vi "Pre Launch Init.vi"(11 "Test Manager in":refnum<class "Test Manager.lvclass">) -> (0 "error out":errorcluster, 3 "Test Manager out":refnum<class "Test Manager.lvclass">)   [LabVIEW 2020, in "Test Manager.lvlib" / "Test Manager.lvclass"]
doc: "Sends a high priority message to it's self to notify the monitor that it's spawned. If it's in the runtime environment, this message is never sent, meaning the monitor will never spawn\n\nCopyright: MGI\n\nAuthored by Derek Trepanier\nsupport@mooregoodideas.com\nwww.mooregoodideas.com\n\nCopyright (c) 2014, Moore Good Ideas, Inc.\n\nAll rights reserved.\n\nRedistribution and use in source and binary forms, with or without modification, are permitted provided that the following conditions are met:\n\n * Redistributions of source code must retain the above copyright notice, this list of conditions and the following disclaimer.\n * Redistributions in binary form must reproduce the above copyright notice, this list of conditions and the following disclaimer in the documentation and/or other materials provided with the distribution.\n * Neither the name of Moore Good Ideas, Inc. nor the names of its contributors may be used to endorse or promote products derived from this software without specific prior written permission.\n\nTHIS SOFTWARE IS PROVIDED BY THE COPYRIGHT HOLDERS AND CONTRIBUTORS \"AS IS\" AND ANY EXPRESS OR IMPLIED WARRANTIES, INCLUDING, BUT NOT LIMITED TO, THE IMPLIED WARRANTIES OF MERCHANTABILITY AND FITNESS FOR A PARTICULAR PURPOSE ARE DISCLAIMED. IN NO EVENT SHALL THE COPYRIGHT OWNER OR CONTRIBUTORS BE LIABLE FOR ANY DIRECT, INDIRECT, INCIDENTAL, SPECIAL, EXEMPLARY, OR CONSEQUENTIAL DAMAGES (INCLUDING, BUT NOT LIMITED TO, PROCUREMENT OF SUBSTITUTE GOODS OR SERVICES; LOSS OF USE, DATA, OR PROFITS; OR BUSINESS INTERRUPTION) HOWEVER CAUSED AND ON ANY THEORY OF LIABILITY, WHETHER IN CONTRACT, STRICT LIABILITY, OR TORT (INCLUDING NEGLIGENCE OR OTHERWISE) ARISING IN ANY WAY OUT OF THE USE OF THIS SOFTWARE, EVEN IF ADVISED OF THE POSSIBILITY OF SUCH DAMAGE."
uses:
  Test Manager.lvclass
  _Abstract Classes/Testing Asset/Testing Asset.lvclass
  _Abstract Classes/Test/Test.lvclass
  Test Manager.lvclass/Test Manager.ctl
  <vilib>/MGI/Monitored Actor/Monitored Actor/Monitored Actor/Monitored Actor.lvclass
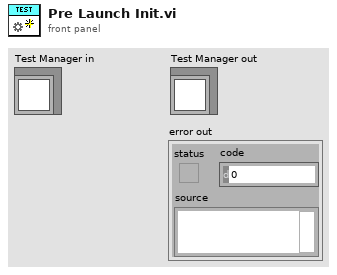
[diagram p1: front panel]
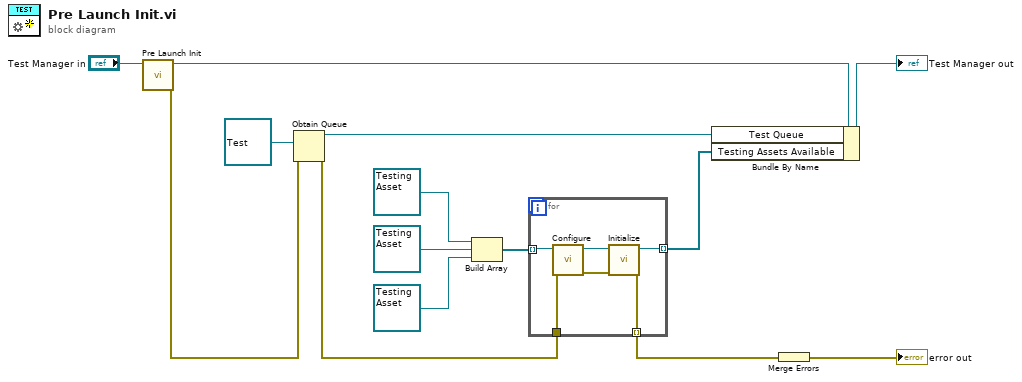
[diagram p0: block diagram]
diagram:
  n1 = call-parent "Pre Launch Init.vi"("Monitored Actor in"="Test Manager in") -> ("error out"=w10:errorcluster, "Monitored Actor out"=w12:refnum<class "Test Manager.lvclass">)  [unwired: 9 in]
  n2 = Obtain Queue(element data type=refnum<class "Test.lvclass"> refnum ("Test Manager.lvlib:Test.lvclass"), error in (no error)=w10) -> (queue out=w8:refnum<queue>, error out=w3:errorcluster)  [unwired: 3 in, 1 out]
  n3 = Build Array(refnum<class "Testing Asset.lvclass"> refnum ("Test Manager.lvlib:Testing Asset.lvclass"), refnum<class "Testing Asset.lvclass"> refnum ("Test Manager.lvlib:Testing Asset.lvclass"), refnum<class "Testing Asset.lvclass"> refnum ("Test Manager.lvlib:Testing Asset.lvclass")) -> (w4:refnum<class "Testing Asset.lvclass">[])
  n4 = for {
    tunnel: w4 -> [w19] mode=indexing
    tunnel: w3 -> [w17]
    tunnel: [w16] -> w2 mode=indexing
    tunnel: [w15] -> w1 mode=indexing
    n5 = call-dynamic "Configure.vi"("error in (no error)"=w17, "Testing Asset in"=w19) -> ("error out"=w18:errorcluster, "Testing Asset out"=w20:refnum<class "Testing Asset.lvclass">)  [unwired: 8 in]
    n6 = call-dynamic "Initialize.vi"("error in (no error)"=w18, "Testing Asset in"=w20) -> ("error out"=w16:errorcluster, "Testing Asset out"=w15:refnum<class "Testing Asset.lvclass">)  [unwired: 8 in]
  }
  n7 = Bundle By Name(cluster=w12, "Test Queue"=w8, "Testing Assets Available"=w1) -> (→"Test Manager out":refnum<class "Test Manager.lvclass">)
  n8 = Merge Errors(w2) -> (→"error out":errorcluster)
